vi "File_SetupTDMS.vi"(8 "error in (no error)":errorcluster, 11 "File in":refnum<class "File.lvclass">) -> (0 "error out":errorcluster, 3 "File out":refnum<class "File.lvclass">)   [LabVIEW 2024, in "File.lvclass"]
doc: "Creates the TDMS file as defined in the class."
uses:
  File.lvclass
  File.lvclass/File.ctl
  Group/Group.lvclass
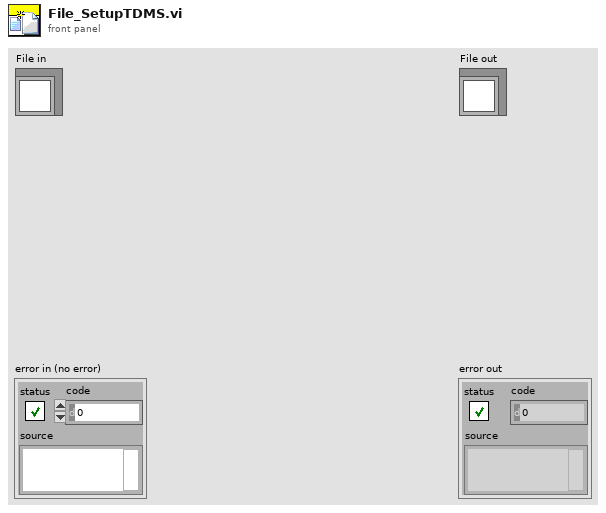
[diagram p1: front panel]
types:
  T1 = enum16{"open", "open or create", "create or replace", "create", "open (read-only)"}
  T2 = typedef "Meta Data.ctl" = cluster{"Key":string, "Value":string}
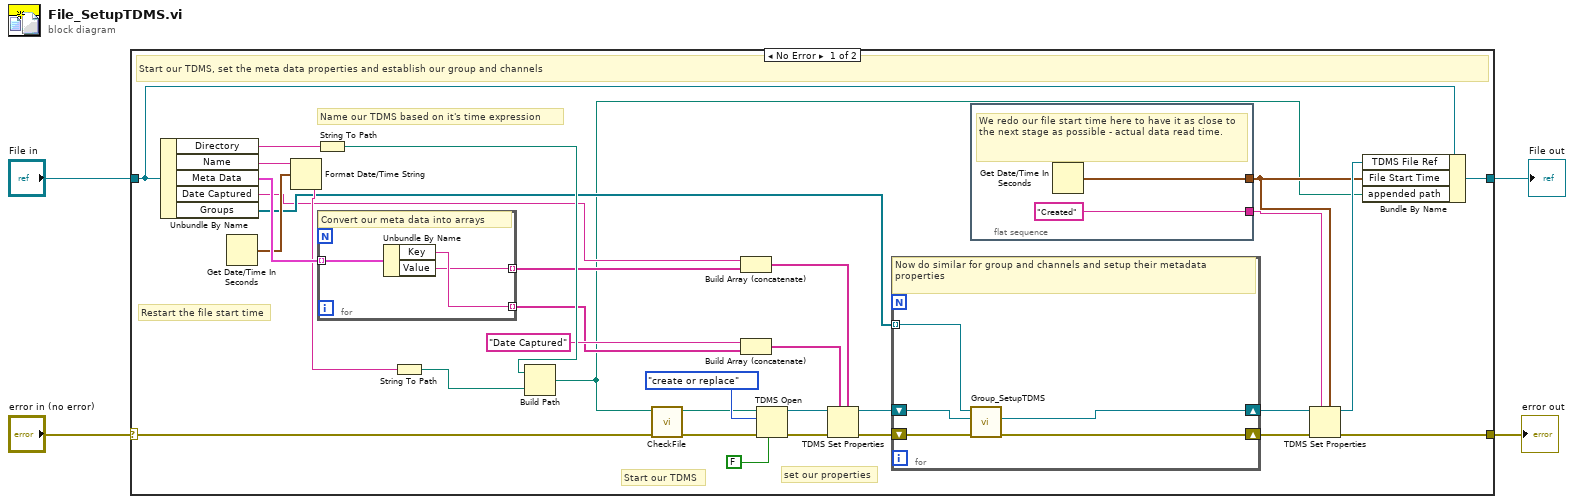
[diagram p0: block diagram]
diagram:
  n1 = case shown="No Error" "error in (no error)" {
    selector: "error in (no error)" -> [w5 w48]
    tunnel: [w23 w48] -> w3
    tunnel: [w18 w47] -> w1
    tunnel: "File in" -> [w21 w47]
    frame No Error {
      # "set our properties"
      # "Name our TDMS based on it's time expression"
      # "Start our TDMS"
      # "Restart the file start time"
      # "Start our TDMS, set the meta data properties and establish our group and channels"
      n2 = Unbundle By Name(w21) -> ("Directory"=w28:string, "Name"=w32:string, "Meta Data"=w34:T2[], "Date Captured"=w13:string, "Groups"=w27:refnum<class "Group.lvclass">[])
      n3 = Get Date/Time In Seconds() -> (seconds since 1Jan1904=w33:timestamp)
      n4 = Format Date/Time String(time format string (%c)=w32, seconds (now)=w33) -> (date/time string=w29:string)  [unwired: 1 in]
      n5 = String To Path(string=w28) -> (path=w31:path)
      n6 = for {
        tunnel: w34 -> [w46] mode=indexing
        tunnel: [w45] -> w15 mode=indexing
        tunnel: [w44] -> w12 mode=indexing
        # "Convert our meta data into arrays"
        n7 = Unbundle By Name(w46) -> ("Key"=w45:string, "Value"=w44:string)
      }
      n8 = String To Path(string=w29) -> (path=w30:path)
      n9 = Build Path(base path=w31, name or relative path=w30) -> (appended path=w8:path)
      n10 = call "CheckFile.vi"("error in (no error)"=w5, "path"=w8) -> ("error out"=w6:errorcluster, "path out"=w7:path)  [unwired: 8 in]
      n11 = Build Array (concatenate)(w13, w12) -> (w11:string[])
      n12 = Build Array (concatenate)("Date Captured", w15) -> (w14:string[])
      n13 = TDMS Open(6:FALSE ("disable buffering? (T)"), 8:w6, 10:T1."create or replace" ("operation (0:open)"), 11:w7) -> (0:w9:errorcluster, 3:w10:refnum<k34>)  [unwired: 3 in]
      n14 = TDMS Set Properties(5:w11, 7:w14, 8:w9, 11:w10) -> (0:w26:errorcluster, 3:w25:refnum<k34>)  [unwired: 1 in, 3 out]
      n15 = for {
        tunnel: w27 -> [w43] mode=indexing
        shift-right: [w40] -> w24
        shift-left: w26 -> [w41]
        shift-right: [w39] -> w17
        shift-left: w25 -> [w42]
        # "Now do similar for group and channels and setup their metadata properties"
        n16 = call-dynamic "Group_SetupTDMS.vi"("error in (no error)"=w41, "tdms file in"=w42, "Group in"=w43) -> ("error out"=w40:errorcluster, "tdms file out"=w39:refnum<k34>)  [unwired: 6 in, 1 out]
      }
      n17 = flat-sequence {
        tunnel: [w38] -> w19
        tunnel: ["Created" ("Name")] -> w22
        frame #0 {
          # "We redo our file start time here to have it as close to the next stage as possible - actual data read time."
          n18 = Get Date/Time In Seconds() -> (seconds since 1Jan1904=w38:timestamp)
        }
      }
      n19 = TDMS Set Properties(5:w19, 7:w22, 8:w24, 11:w17) -> (0:w23:errorcluster, 3:w20:refnum<k34>)  [unwired: 1 in, 3 out]
      n20 = Bundle By Name(cluster=w21, "TDMS File Ref"=w20, "File Start Time"=w19, "appended path"=w8) -> (w18:refnum<class "File.lvclass">)
    }
    frame Error {
    }
  }
  "error out" <- w3
  "File out" <- w1
